vi "MSEditor_DeleteStringLeadingSpace.vi"(0 "string in":string) -> (1 "string after leading space":string, 2 "offset past leading space":i32)   [LabVIEW 2018]
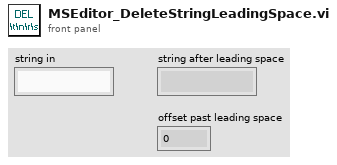
[diagram p1: front panel]
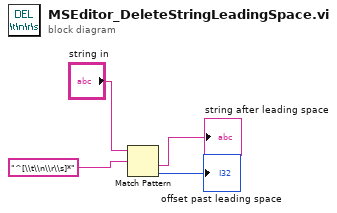
[diagram p0: block diagram]
diagram:
  n1 = Match Pattern(string="string in", regular expression="^[\\t\\n\\r\\s]*") -> (after substring=→"string after leading space":string, offset past match=→"offset past leading space":i32)  [unwired: 1 in, 2 out]
